vi "FromRepo.vi"(8 "error in":errorcluster, 9 "from repo cluster":T2, 10 "repository in":refnum<class "NISE_CEF_Repository.lvclass">, 11 "node in":refnum<class "TimingSource.lvclass">) -> (0 "error out":errorcluster, 2 "repository out":refnum<class "NISE_CEF_Repository.lvclass">, 3 "node":T1)   [LabVIEW 2015, in "TimingSource.lvclass"]
doc: "Grabs information from the Repo and stores it in the nodes."
uses:
  TimingSource.lvclass
  <vilib>/NI/Configuration Framework/Repository/NISE_CEF_Repository.lvclass
  <vilib>/NI/Configuration Framework/Node/FromRepoCluster.ctl
  <vilib>/NI/Configuration Framework/Node/NodeRef.ctl
  <vilib>/NI/Configuration Framework/Node/NISE_CEF_Node.lvclass
  CustomDeviceRepo/CustomDeviceRepo.lvclass
  CustomDeviceRepo/CustomDeviceRepo.lvclass/CustomDeviceRepo.ctl
  TimingSource.lvclass/TimingSource.ctl
  CustomDeviceRepo/Read Timing Source Properties.vi
  Write Timing Source Properties.vi
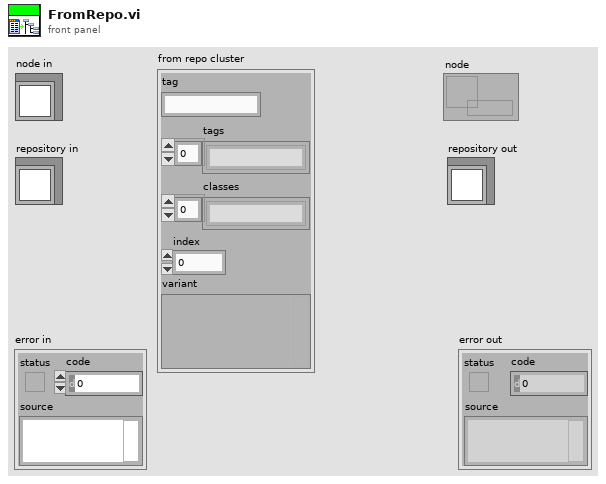
[diagram p1: front panel]
types:
  T1 = typedef "NISE_CEF_Node.lvclass/NodeRef.ctl" = refnum<data-value>
  T2 = typedef "NISE_CEF_Node.lvclass/FromRepoCluster.ctl" = cluster{"tag":string, "tags":string[], "classes":string[], "index":i32, "variant":variant}
  T3 = typedef "Timing Source Properties.ctl" = cluster{"Has Timing Source Capability":bool, "Source Distribution":T4}
  T4 = typedef "Source Distribution for TimingSource.ctl" = cluster{"Supported Target":T5, "Source":T6, "Real Time System Destination":string, "Version":string}[]
  T5 = typedef "Target.ctl" = enum16{"All", "Pharlap", "VxWorks", "Windows", "Linux_32_ARM", "Linux_x64", "PharlapWindows", "PharlapVxWorks", "VxWorksWindows"}
  T6 = typedef "Path Cluster.ctl" = cluster{"Path":path, "Path Type":enum16{"Absolute", "To Base", "To Common Doc Dir", "To Application Data Dir"}}
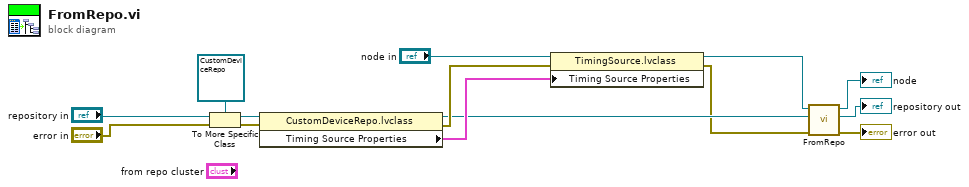
[diagram p0: block diagram]
diagram:
  n1 = To More Specific Class(target class=refnum<class "CustomDeviceRepo.lvclass"> refnum, reference="repository in", error in="error in") -> (specific class reference=w8:refnum<class "CustomDeviceRepo.lvclass">, error out=w9:errorcluster)
  n2 = property class="CustomDeviceRepo.lvclass"(reference=w8, error in=w9) -> (reference out=w3:refnum<class "CustomDeviceRepo.lvclass">, error out=w11:errorcluster, "Timing Source Properties"=w10:T3)
  n3 = property class="TimingSource.lvclass"(reference="node in", error in=w11, "Timing Source Properties"=w10) -> (reference out=w2:refnum<class "TimingSource.lvclass">, error out=w1:errorcluster)
  n4 = call-parent "FromRepo.vi"("error in"=w1, "repository in"=w3, "node in"=w2) -> ("error out"=→"error out":errorcluster, "repository out"=→"repository out":refnum<class "NISE_CEF_Repository.lvclass">, "node"=→"node":T1)  [unwired: 6 in]
